vi "Change Bit (I64).vi"(9 "Value":bool=TRUE, 10 "Bit":u8, 11 "Number":i64 format="%.0x") -> (3 "Number Out":i64 format="%.0x")   [LabVIEW 2019, in "Bits.lvlib"]
uses:
  Bits.lvlib
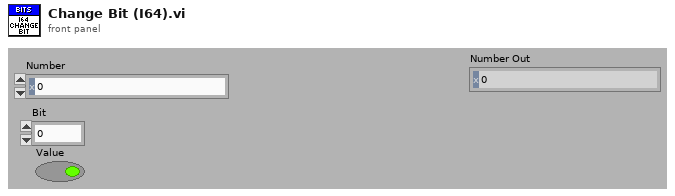
[diagram p1: front panel]
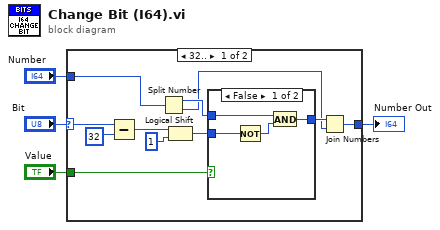
[diagram p0: block diagram]
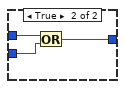
[diagram p2: hidden frame]
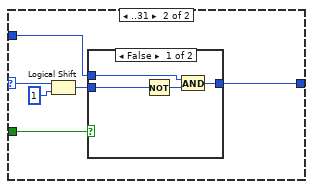
[diagram p3: hidden frame]
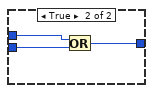
[diagram p4: hidden frame]
diagram:
  n1 = case shown="32.." "Bit" {
    selector: "Bit" -> [w13 w27]
    tunnel: "Number" -> [w9 w26]
    tunnel: [w8 w24] -> w2
    tunnel: "Value" -> [w5 w23]
    frame 32.. {
      n2 = Subtract(x=w13, y=u8 32 ("x")) -> (x-y=w14:u8)
      n3 = Split Number(x=w9) -> (hi(x)=w12:u32, lo(x)=w10:u32)
      n4 = Logical Shift(y=w14, x=u32 1) -> (x << y=w7:u32)
      n5 = case shown="False" w5 {
        tunnel: w12 -> [w19 w22]
        tunnel: [w16 w21] -> w11
        tunnel: w7 -> [w18 w20]
        frame False {
          n6 = Not(x=w18) -> (.not. x?=w17:u32)
          n7 = And(x=w19, y=w17) -> (x .and. y?=w16:u32)
        }
        frame True {
          n8 = Or(x=w22, y=w20) -> (x .or. y?=w21:u32)
        }
      }
      n9 = Join Numbers(hi=w11, lo=w10) -> ((hi.lo)=w8:u64)
    }
    frame ..31 {
      n10 = Logical Shift(y=w27, x=u32 1) -> (x << y=w25:u32)
      n11 = case shown="False" w23 {
        tunnel: w26 -> [w32 w35]
        tunnel: [w29 w34] -> w24
        tunnel: w25 -> [w31 w33]
        frame False {
          n12 = Not(x=w31) -> (.not. x?=w30:u32)
          n13 = And(x=w32, y=w30) -> (x .and. y?=w29:i64)
        }
        frame True {
          n14 = Or(x=w35, y=w33) -> (x .or. y?=w34:i64)
        }
      }
    }
  }
  "Number Out" <- w2
